vi "RT.vi"() -> ()   [LabVIEW 2015]
uses:
  <vilib>/FPGAPlugInAG/cRIO-9068/niLvFpga_Open_cRIO-9068.vi
  <vilib>/rvi/interface/common/dynamic/niFpgaDynamicAddResources.vi
  <vilib>/rvi/Analysis/host/Private/Sample Rate To Loop Time (ticks).vi
  <vilib>/Utility/error.llb/Error Cluster From Error Code.vi
  <vilib>/rvi/errors/niLvFpgaAdjustHostInterfaceError.vi
  <vilib>/FPGAPlugInAG/Dynamic/niLvFpga_Close_Dynamic.vi
  <vilib>/rvi/interface/nirviOpenFPGA/nirviOpenFPGA.xnode
  FPGA Bitfiles/UntitledProject2_FPGATarget_Untitled2_wGPC87C8Mk8.lvbitx
  FPGA.vi
  <vilib>/rvi/interface/nirviReadWriteControl/nirviReadWriteControl.xnode
  <vilib>/rvi/interface/nirviMethod/nirviMethod.xnode
  <vilib>/rvi/interface/nirviCloseFPGA/nirviCloseFPGA.xnode
  <vilib>/rvi/Analysis/host/Public/NI_FpgaMspHost.lvlib
  <vilib>/FPGAPlugInAG/Dynamic/niLvFpga_ReadFifo_Dynamic.vi
  <vilib>/rvi/errors/niLvFpgaMergeErrorWithErrorCode.vi
  NiFpgaLv.dll
  <vilib>/rvi/interface/Simulation/niFpgaSimulationCallBeginRW.vi
panel:
  in  "y":fxp<+/-,16,1>
  out "actual sample rate (S/s)":dbl format="%#_6p"
  out "error out":errorcluster
  out "Waveform Chart":waveform(dbl)(graph)
  in  "stop":bool
  in  "sample rate (S/s)":dbl format="%#_6p"
  in  "frequency (Hz)":dbl format="%#_6p"
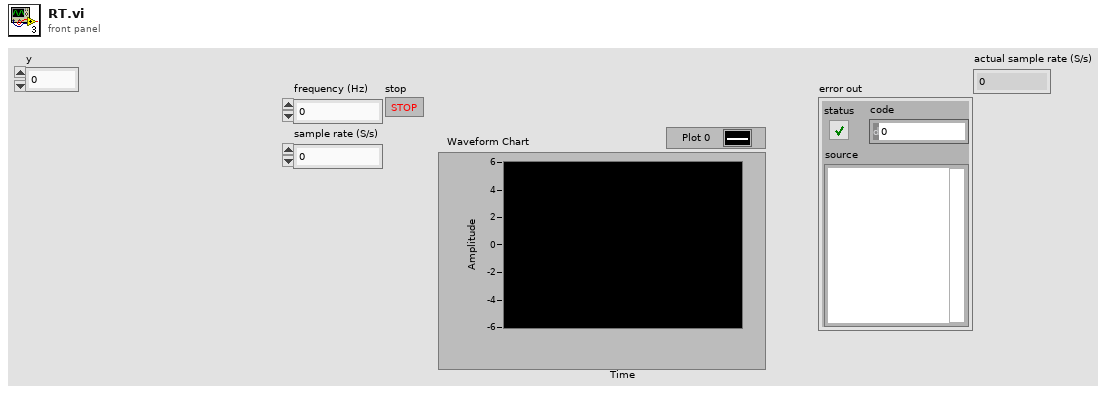
[diagram p1: front panel]
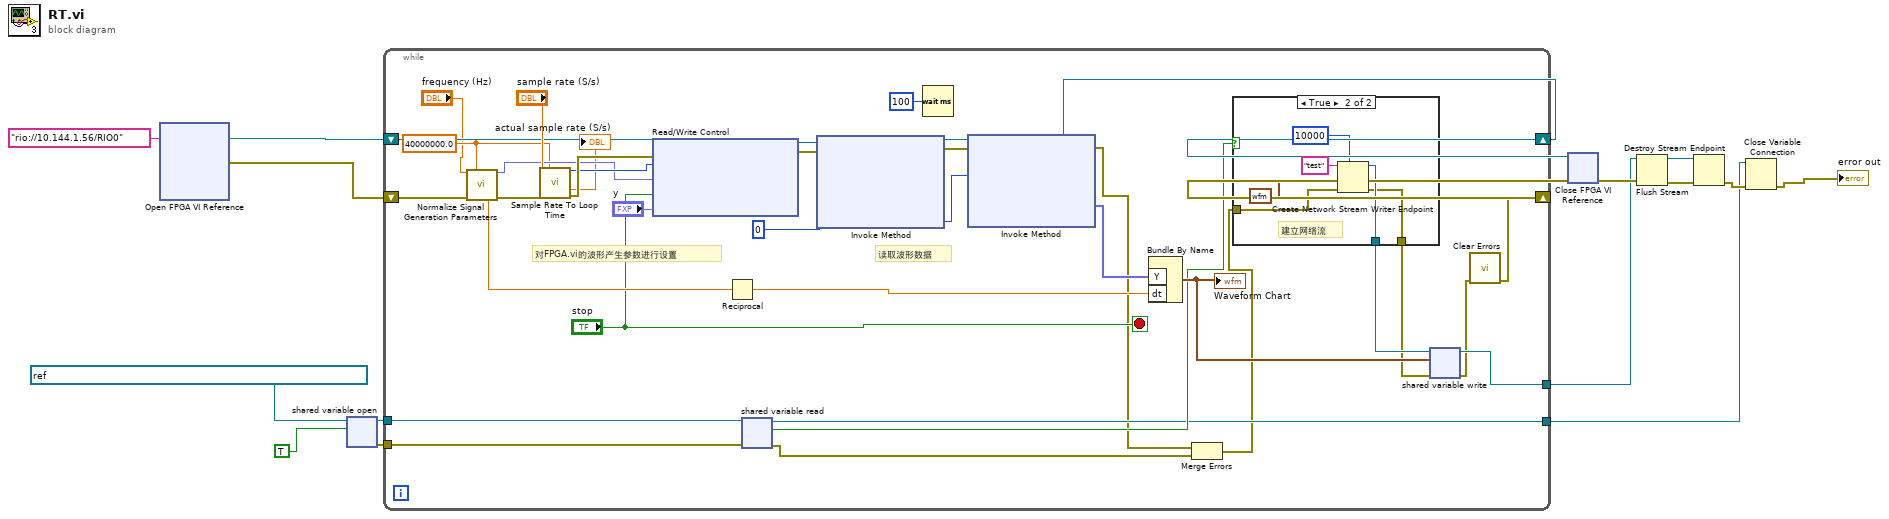
[diagram p0: block diagram]
diagram:
  n1 = xnode "Open FPGA VI Reference"("resource name"=tag "rio://10.144.1.56/RIO0") -> ("FPGA VI Reference Out"=w2:refnum<k20>, "error out"=w16:errorcluster)  [unwired: 1 in]
  n2 = shared-variable-open(refnum<k21> "ni.var.psp://ni-crio-9068-18dd4b9/Untitled Library 1/signal" ("shared variable refnum in"), TRUE) -> (w6:refnum<k21>, w7:errorcluster)  [unwired: 2 in]
  n3 = while {
    shift-right: [w40] -> w15
    shift-left: w2 -> [w49]
    shift-right: [w25] -> w14
    shift-left: w16 -> [w51]
    tunnel: [w29] -> w12
    tunnel: w7 -> [w24]
    tunnel: w6 -> [w23]
    tunnel: [w21] -> w3
    stop <- "stop" stop-if-true
    w45 = 40000000.0 ("FPGA clock rate (Hz)")
    # "读取波形数据"
    # "对FPGA.vi的波形产生参数进行设置"
    n4 = call <vilib>:"Normalize Signal Generation Parameters.vi"("frequency (Hz)"="frequency (Hz)", "FPGA clock rate (Hz)"=w45, "error in (no error)"=w51) -> ("frequency (periods/tick)"=w46:fxp<+,32,0>, "actual frequency (Hz)"=w44:dbl, "error out"=w50:errorcluster)  [unwired: 7 in, 3 out]
    n5 = call-poly <vilib>:"Sample Rate To Loop Time.vi"("sample rate (S/s)"="sample rate (S/s)", "FPGA clock rate (Hz)"=w45, "error in (no error)"=w50) -> ("count (ticks/S)"=w47:u32, "actual sample rate (S/s)"=→"actual sample rate (S/s)":dbl, "error out"=w48:errorcluster)  [unwired: 10 in]
    n6 = xnode "Read/Write Control"("FPGA VI Reference In"=w49, "error in"=w48, "Sample Rate"=w47, "frequency (periods/tick)"=w46, "stop"="stop", "y"="y") -> ("FPGA VI Reference Out"=w36:refnum<k20>, "error out"=w35:errorcluster)
    n7 = Reciprocal(x=w44) -> (1/x=w42:dbl)
    n8 = shared-variable-read(w23, w24) -> (w21:refnum<k21>, w19:errorcluster, w22:bool)  [unwired: 1 out]
    n9 = xnode "Invoke Method"("FPGA VI Reference In"=w36, "error in"=w35, "Number of Elements"=u32 0) -> ("FPGA VI Reference Out"=w38:refnum<k20>, "error out"=w37:errorcluster, "Elements Remaining"=w33:u32)  [unwired: 1 in, 1 out]
    n10 = Wait (ms)(milliseconds to wait=u32 100) -> ()  [unwired: 1 out]
    n11 = xnode "Invoke Method"("FPGA VI Reference In"=w38, "error in"=w37, "Number of Elements"=w33) -> ("FPGA VI Reference Out"=w40:refnum<k20>, "error out"=w20:errorcluster, "Data"=w43:fxp<+/-,16,16>[])  [unwired: 1 in, 1 out]
    n12 = Bundle By Name("Y"=w43, "dt"=w42) -> (w30:waveform(dbl))  [unwired: 1 in]
    "Waveform Chart" <- w30
    n13 = Merge Errors(w20, w19) -> (w18:errorcluster)
    n14 = case shown="True" w22 {
      tunnel: [_ w55] -> w28
      tunnel: [_ w54] -> w27
      tunnel: w18 -> [_ w53]
      frame False {
      }
      frame True {
        # "建立网络流"
        n15 = Create Network Stream Writer Endpoint(7:10000 ("writer buffer size"), 8:w53, 9:waveform(dbl) {"t0"=timestamp(0 s since 1904-01-01), "dt"=1.0, "Y"=[]} ("Waveform"), 11:"test" ("writer name")) -> (0:w54:errorcluster, 3:w55:refnum<k21>)  [unwired: 3 in]
      }
    }
    n16 = shared-variable-write(w28, w27, w30) -> (w29:refnum<k21>, w26:errorcluster)  [unwired: 1 in, 1 out]
    n17 = call <vilib>:"Clear Errors.vi"("error in (no error)"=w26) -> ("error out"=w25:errorcluster)  [unwired: 5 in, 1 out]
  }
  n18 = xnode "Close FPGA VI Reference"("FPGA VI Reference In"=w15, "error in"=w14) -> ("error out"=w13:errorcluster)
  n19 = Flush Stream(8:w13, 11:w12) -> (0:w11:errorcluster, 3:w10:refnum<k21>)  [unwired: 2 in, 1 out]
  n20 = Destroy Stream Endpoint(8:w11, 11:w10) -> (0:w5:errorcluster)
  n21 = Close Variable Connection(8:w5, 11:w3) -> (0:→"error out":errorcluster)
